vi "_logging_data_string_to_log_string.vi"(7 "Force binary format (F)":bool, 8 "error in":errorcluster caption="error in (no error)", 10 "Raw string to log":string, 11 "VISA resource name":refnum<visa-resource-name>) -> (0 "error out":errorcluster, 2 "Result log string":string, 3 "VISA resource name out":refnum<visa-resource-name>)   [LabVIEW 2020, in "Rohde&Schwarz RTx Oscilloscopes.lvlib" / "rsidr_core.lvlib"]
uses:
  rsidr_core.lvlib
  _type_Logging_Parameter.ctl
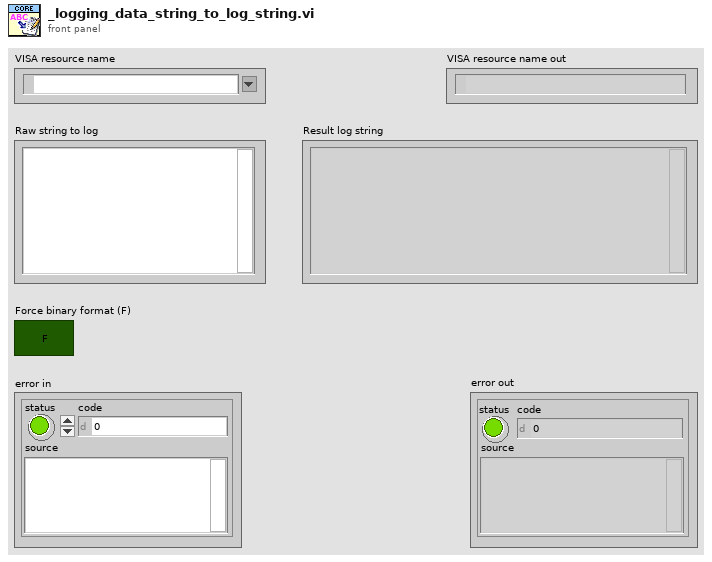
[diagram p1: front panel]
types:
  T1 = typedef "Rohde&Schwarz RTx Oscilloscopes.lvlib/rsidr_core.lvlib/_type_Logging_Parameter.ctl" = enum16{"Type (String)", "SessionAlias(String)", "FormatString (String)", "UDPconectionID (I32)", "UDPlocalPort (I32)", "UDPremotePort (I32)", "UDPremoteHost (String)", "FILEmode (I32)", "FILEpath (String)", "FILEopenID (I32)", "DataMaxLogLen (I32)"}
  T2 = typedef "Rohde&Schwarz RTx Oscilloscopes.lvlib/rsidr_core.lvlib/type_Session_Data.ctl" = cluster{"IDN string":string, "Instrument FW":string, "Instr type":string, "Instr type for err. msg.":string, "Installed Options":string[], "Ignore Error Messages":string, "Logging params":variant, "OPC Timeout":i32, "VISA Timeout":i32, "STB Poll VISA Timeout":i32, "Additional Flags":i32, "Wait Before Read":i32, "Wait Before Write":i32, "Option String Flags":i32, "IO Segment Size":i64, "VISA Access Mode":T3, "Interface Type":T4, "OPC Wait Mode":T5, "Bin Float Number  Format":T6, "Bin Integer Number Format":T7, "Simulate":bool, "VXIcapable":bool, "Duplicate Session":bool, "Add LF to Write":bool, "Logging":bool, "Fast Sweep":bool, "Query Instrument Status":bool, "Check Range":bool, "Check Options":bool, "OPC-sync Attr Writes":bool, "OPC-sync Attr Queries":bool}
  T3 = typedef "Rohde&Schwarz RTx Oscilloscopes.lvlib/rsidr_core.lvlib/type_VisaAccessMode.ctl" = u16
  T4 = typedef "Rohde&Schwarz RTx Oscilloscopes.lvlib/rsidr_core.lvlib/type_InterfaceType.ctl" = enum16{"Unknown", "GPIB", "VXI", "GPIB_VXI", "ASRL", "PXI", "TCPIP", "USB", "SOCKET"}
  T5 = typedef "Rohde&Schwarz RTx Oscilloscopes.lvlib/rsidr_core.lvlib/type_OPC_Wait_Mode.ctl" = enum16{"STBpolling", "STBpollingSlow", "STBpollingSuperSlow", "ServiceRequest", "OPCquery"}
  T6 = typedef "Rohde&Schwarz RTx Oscilloscopes.lvlib/rsidr_core.lvlib/type_Binary_Float_Number_Format.ctl" = enum16{"Float_4_Bytes_Swapped", "Float_4_Bytes", "Double_8_Bytes_Swapped", "Double_8_Bytes"}
  T7 = typedef "Rohde&Schwarz RTx Oscilloscopes.lvlib/rsidr_core.lvlib/type_Binary_Integer_Number_Format.ctl" = enum16{"Int32_4_Bytes_Swapped", "Int32_4 Bytes", "Int16_2_Bytes_Swapped", "Int16_2_Bytes"}
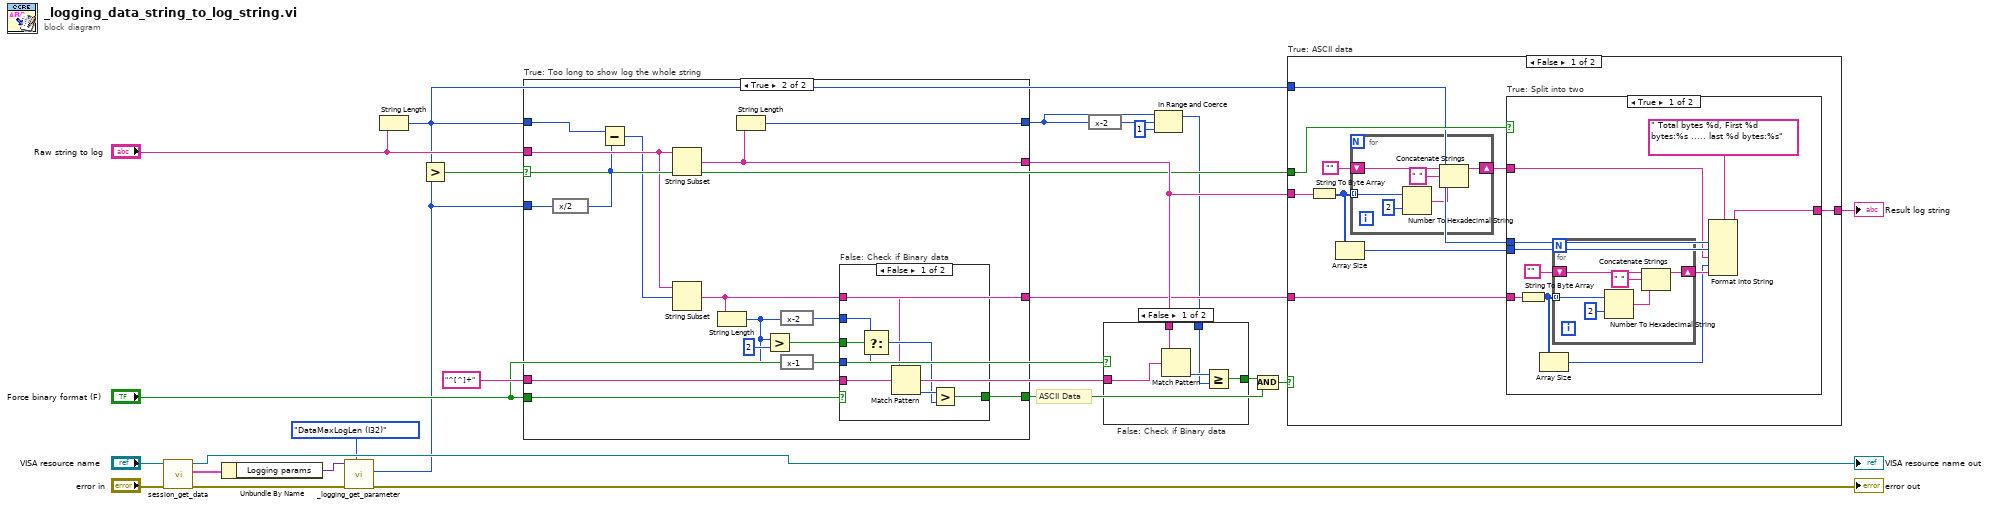
[diagram p0: block diagram]
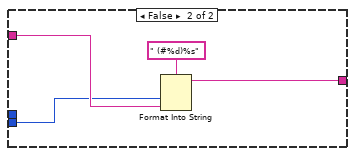
[diagram p3: hidden frame]
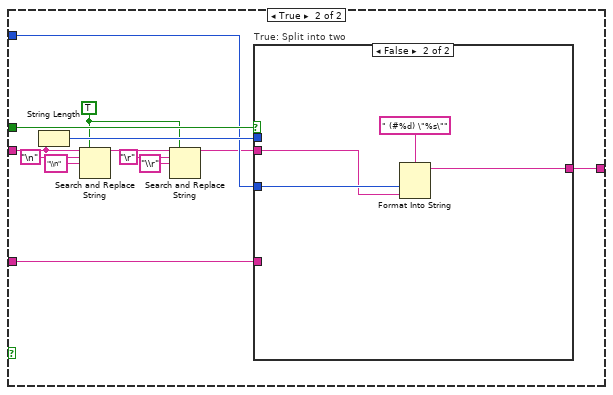
[diagram p4: hidden frame]
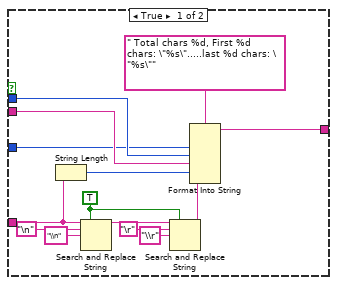
[diagram p5: hidden frame]
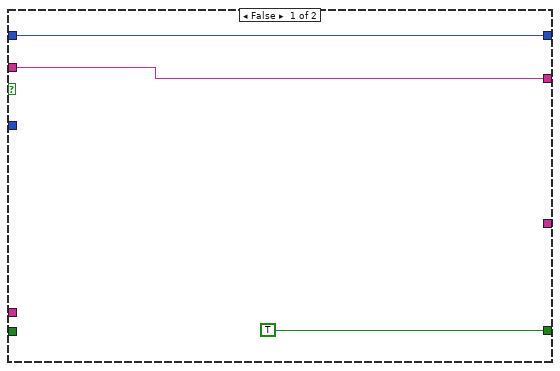
[diagram p6: hidden frame]
diagram:
  w22 = "^[^]+" ("regular expression")
  # "ASCII Data"
  n1 = call "session_get_data.vi"("error in"="error in", "VISA resource name"="VISA resource name") -> ("error out"=w6:errorcluster, "Session User Data out"=w10:T2, "VISA resource name out"=→"VISA resource name out":refnum<visa-resource-name>)  [unwired: 6 in, 1 out]
  n2 = Unbundle By Name(w10) -> ("Logging params"=w9:variant)
  n3 = call "_logging_get_parameter.vi"("Logging Parameter"=_type_Logging_Parameter."DataMaxLogLen (I32)", "error in"=w6, "Logging params in"=w9) -> ("error out"=→"error out":errorcluster, "Int32 parameter out"=w2:i32)  [unwired: 4 in, 3 out]
  n4 = String Length(string="Raw string to log") -> (length=w18:i32)
  n5 = Greater?(x=w18, y=w2) -> (0:w20:bool)
  n6 = case "True: Too long to show log the whole string" shown="True" w20 {
    tunnel: "Raw string to log" -> [w27 w42]
    tunnel: w2 -> [_ w43]
    tunnel: w18 -> [w26 w41]
    tunnel: [w27 w38] -> w23
    tunnel: [w26 w39] -> w11
    tunnel: [_ w28] -> w21
    tunnel: w22 -> [_ w32]
    tunnel: [TRUE w31] -> w17
    tunnel: "Force binary format (F)" -> [_ w29]
    frame False {
    }
    frame True {
      n7 = expression code="x/2"(w43) -> (w30:i32)
      n8 = Subtract(x=w41, y=w30) -> (x-y=w40:i32)
      n9 = String Subset(string=w42, length (rest)=w30) -> (substring=w38:string)  [unwired: 1 in]
      n10 = String Subset(string=w42, offset (0)=w40) -> (substring=w28:string)  [unwired: 1 in]
      n11 = String Length(string=w28) -> (length=w33:i32)
      n12 = String Length(string=w38) -> (length=w39:i32)
      n13 = Greater?(x=w33, y=2) -> (0:w36:bool)
      n14 = expression code="x-2"(w33) -> (w35:i32)
      n15 = expression code="x-1"(w33) -> (w34:i32)
      n16 = case "False: Check if Binary data" shown="False" w29 {
        tunnel: w36 -> [w51 _]
        tunnel: w35 -> [w50 _]
        tunnel: w34 -> [w49 _]
        tunnel: w32 -> [w48 _]
        tunnel: [w45 _] -> w31
        tunnel: w28 -> [w44 _]
        frame False {
          n17 = Select(t=w50, s=w51, f=w49) -> (s? t:f=w46:i32)
          n18 = Match Pattern(string=w44, regular expression=w48) -> (offset past match=w47:i32)  [unwired: 1 in, 3 out]
          n19 = Greater?(x=w47, y=w46) -> (0:w45:bool)
        }
        frame True {
        }
      }
    }
  }
  n20 = expression code="x-2"(w11) -> (w14:i32)
  n21 = In Range and Coerce(upper limit=w11, x=w14, lower limit=1) -> (coerced(x)=w13:i32)  [unwired: 1 out]
  n22 = case "False: Check if Binary data" shown="False" "Force binary format (F)" {
    tunnel: w13 -> [w55 _]
    tunnel: w23 -> [w54 _]
    tunnel: w22 -> [w53 _]
    tunnel: [w52 _] -> w16
    frame False {
      n23 = Match Pattern(string=w54, regular expression=w53) -> (offset past match=w56:i32)  [unwired: 1 in, 3 out]
      n24 = Greater Or Equal?(x=w56, y=w55) -> (x >= y?=w52:bool)
    }
    frame True {
    }
  }
  n25 = And(x=w16, y=w17) -> (x .and. y?=w15:bool)
  n26 = case "True: ASCII data" shown="False" w15 {
    tunnel: w23 -> [w64 w100]
    tunnel: w21 -> [w63 w101]
    tunnel: w20 -> [w65 w102]
    tunnel: [w58 w98] -> w19
    tunnel: w18 -> [w57 w97]
    frame False {
      n27 = String To Byte Array(string=w64) -> (unsigned byte array=w59:u8[])
      n28 = Array Size(array=w59) -> (size(s)=w60:i32)
      n29 = for {
        tunnel: w59 -> [w71] mode=indexing
        shift-right: [w69] -> w61
        shift-left: "" ("Empty String Constant") -> [w68]
        n30 = Number To Hexadecimal String(1:i16 2 ("width (-)"), 2:w71) -> (0:w66:string)
        n31 = Concatenate Strings(w68, " " ("string"), w66) -> (w69:string)
      }
      n32 = case "True: Split into two" shown="True" w65 {
        tunnel: w63 -> [w80 _]
        tunnel: w61 -> [w74 w90]
        tunnel: w60 -> [w77 w89]
        tunnel: [w76 w88] -> w58
        tunnel: w57 -> [w75 _]
        frame True {
          n33 = String To Byte Array(string=w80) -> (unsigned byte array=w73:u8[])
          n34 = Array Size(array=w73) -> (size(s)=w72:i32)
          n35 = for {
            tunnel: w73 -> [w87] mode=indexing
            shift-right: [w85] -> w78
            shift-left: "" ("Empty String Constant") -> [w84]
            n36 = Number To Hexadecimal String(1:i16 2 ("width (-)"), 2:w87) -> (0:w82:string)
            n37 = Concatenate Strings(w84, " " ("string"), w82) -> (w85:string)
          }
          n38 = Format Into String(format string=" Total bytes %d, First %d bytes:%s ..... last %d bytes:%s", w75, w77, w74, w72, w78) -> (resulting string=w76:string)  [unwired: 2 in, 1 out]
        }
        frame False {
          n39 = Format Into String(format string=" (#%d)%s", w89, w90) -> (resulting string=w88:string)  [unwired: 2 in, 1 out]
        }
      }
    }
    frame True {
      w93 = TRUE ("replace all? (F)")
      n40 = String Length(string=w100) -> (length=w99:i32)
      n41 = Search and Replace String(replace all?=w93, input string=w100, search string="\n" ("Line Feed Constant"), replace string="\\n" ("replace string (\"\")")) -> (result string=w94:string)  [unwired: 4 in, 3 out]
      n42 = Search and Replace String(replace all?=w93, input string=w94, search string="\r" ("Carriage Return Constant"), replace string="\\r" ("replace string (\"\")")) -> (result string=w92:string)  [unwired: 4 in, 3 out]
      n43 = case "True: Split into two" shown="False" w102 {
        tunnel: w101 -> [w114 _]
        tunnel: w92 -> [w112 w119]
        tunnel: w99 -> [w115 w120]
        tunnel: [w113 w121] -> w98
        tunnel: w97 -> [w110 _]
        frame True {
          w107 = TRUE ("replace all? (F)")
          n44 = String Length(string=w114) -> (length=w111:i32)
          n45 = Search and Replace String(replace all?=w107, input string=w114, search string="\n" ("Line Feed Constant"), replace string="\\n" ("replace string (\"\")")) -> (result string=w109:string)  [unwired: 4 in, 3 out]
          n46 = Search and Replace String(replace all?=w107, input string=w109, search string="\r" ("Carriage Return Constant"), replace string="\\r" ("replace string (\"\")")) -> (result string=w108:string)  [unwired: 4 in, 3 out]
          n47 = Format Into String(format string=" Total chars %d, First %d chars: \"%s\".....last %d chars: \"%s\"", w110, w115, w112, w111, w108) -> (resulting string=w113:string)  [unwired: 2 in, 1 out]
        }
        frame False {
          n48 = Format Into String(format string=" (#%d) \"%s\"", w120, w119) -> (resulting string=w121:string)  [unwired: 2 in, 1 out]
        }
      }
    }
  }
  "Result log string" <- w19
